vi "AB_Set_Exclusions.vi"(4 "Exclude dependent shared libraries":bool, 6 "Exclude dependent packed libraries":bool, 8 "error in (no error)":errorcluster, 9 "Disconnect inline subVIs":bool, 10 "Exclusions":T1, 11 "Build in":refnum<class "AB_Build.lvclass">) -> (0 "error out":errorcluster, 3 "Build out":refnum<class "AB_Build.lvclass">)   [LabVIEW 2020]
uses:
  <vilib>/AppBuilder/AB_Classes/Build/AB_Build.lvclass
  <vilib>/AppBuilder/AB_API/common/AB_API Primary Exclusions.ctl
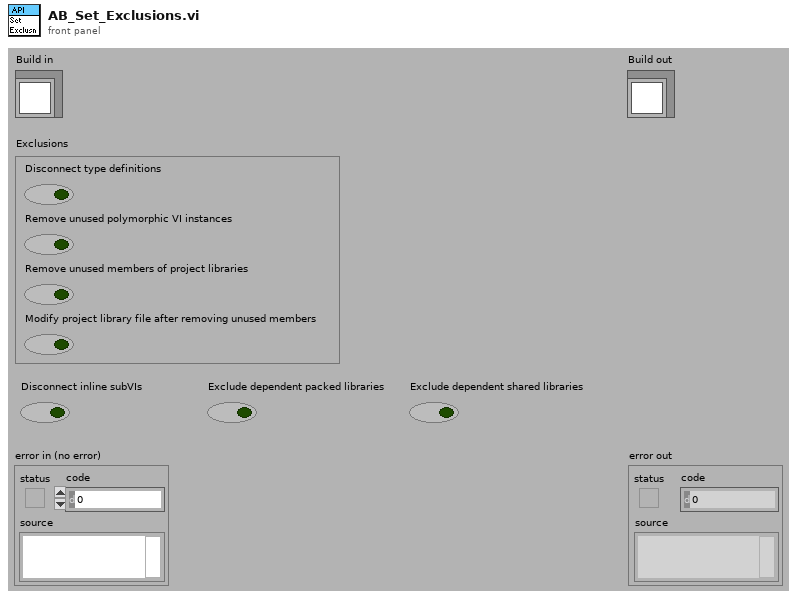
[diagram p1: front panel]
types:
  T1 = typedef "AB_API Primary Exclusions.ctl" = cluster{"Disconnect type definitions":bool, "Remove unused polymorphic VI instances":bool, "Remove unused members of project libraries":bool, "Modify project library file after removing unused members":bool}
  T2 = typedef "AB_Build.ctl" = cluster{"buildSpecName":string, "buildSpecDescription":string, "destinations":refnum<class "AB_Destination.lvclass">[], "exclusionOption":T3, "defaultLanguage":string, "supportedLanguages":string[], "excludedDirectories":path[], "buildContext":refnum<vi>, "buildObject":T4, "preview":bool, "programatic":bool, "progressBarEvents":T5, "userLog_Path":path, "preActionID":string, "preAction_Path":path, "postActionID":string, "postAction_Path":path, "eng_checkForBrokenVIs?":bool, "eng_verboseLinkerErrors?":bool, "localDest_Path":path, "targetDest_Path":path, "removeVIObject":u16, "cache":refnum<class "PreviewCache.lvclass">, "use cache":bool, "previewCache_ID":string, "buildCache_ID":string, "eng_TempLocalDest_Path":path, "eng_collectDependencies?":bool, "versionInfo":cluster{"buildVersion":cluster{"major":u16, "minor":u16, "patch":u16, "build":u16}, "autoIncrement":bool}, "eng_enableVIChecksums":bool}
  T3 = typedef "AB_Exclusion_Option.ctl" = cluster{"typedefs":bool, "polymorphicVIs":bool, "unusedLibraryItems":bool, "modifyLibraryFile":bool, "edit-timeDependencies":bool, "inlineVIs":bool, "dependent PPLs":bool, "dependent DLLs":bool}
  T4 = typedef "ItemRef.ctl" = u64
  T5 = typedef "provcom_ProgressBar_Events.ctl" = cluster{"newJob":refnum<user-event>, "newItem":refnum<user-event>, "errorMsg":T6, "cancel":refnum<user-event>}
  T6 = typedef "mxLvBuildError.ctl" = refnum<user-event>
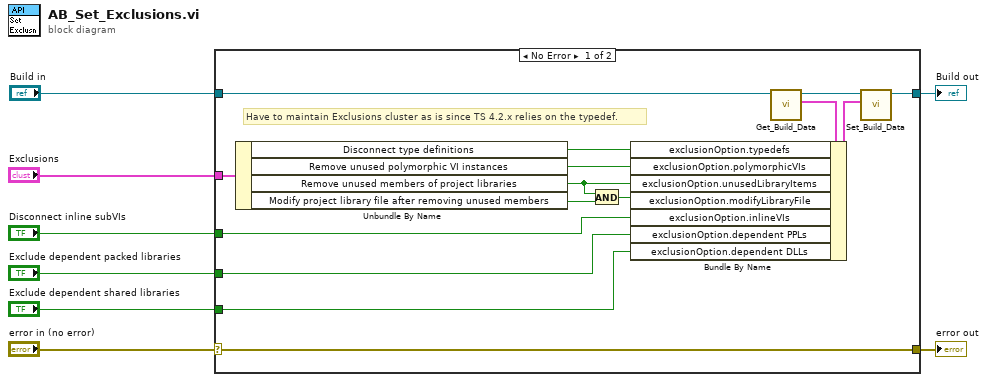
[diagram p0: block diagram]
diagram:
  n1 = case shown="No Error" "error in (no error)" {
    selector: "error in (no error)" -> [w12 w25]
    tunnel: [w12 w25] -> w7
    tunnel: [w13 w24] -> w6
    tunnel: "Build in" -> [w14 w24]
    tunnel: "Exclusions" -> [w15 _]
    tunnel: "Disconnect inline subVIs" -> [w11 _]
    tunnel: "Exclude dependent packed libraries" -> [w10 _]
    tunnel: "Exclude dependent shared libraries" -> [w9 _]
    frame No Error {
      # "Have to maintain Exclusions cluster as is since TS 4.2.x relies on the typedef."
      n2 = Unbundle By Name(w15) -> ("Disconnect type definitions"=w18:bool, "Remove unused polymorphic VI instances"=w19:bool, "Remove unused members of project libraries"=w17:bool, "Modify project library file after removing unused members"=w16:bool)
      n3 = And(x=w17, y=w16) -> (x .and. y?=w20:bool)
      n4 = call <vilib>:"Get_Build_Data.vi"("Class in"=w14) -> ("data"=w23:T2, "Class out"=w21:refnum<class "AB_Build.lvclass">)  [unwired: 1 in, 8 out]
      n5 = Bundle By Name(cluster=w23, "exclusionOption.typedefs"=w18, "exclusionOption.polymorphicVIs"=w19, "exclusionOption.unusedLibraryItems"=w17, "exclusionOption.modifyLibraryFile"=w20, "exclusionOption.inlineVIs"=w11, "exclusionOption.dependent PPLs"=w10, "exclusionOption.dependent DLLs"=w9) -> (w22:T2)
      n6 = call <vilib>:"Set_Build_Data.vi"("data"=w22, "Class in"=w21) -> ("Class out"=w13:refnum<class "AB_Build.lvclass">)  [unwired: 1 in, 8 out]
    }
    frame Error {
    }
  }
  "error out" <- w7
  "Build out" <- w6
